vi "Build.vi"(9 "XYZTheta":dbl[](array[numeric]), 10 "Pattern Coordinates":dbl[][](array[numeric]), 11 "Crosshair Dispense in":refnum<class "Crosshair Dispense.lvclass">) -> (1 "Starting Coordinates":dbl[](array[numeric]), 3 "Crosshair Dispense out":refnum<class "Crosshair Dispense.lvclass">)   [LabVIEW 2019, in "Crosshair Dispense.lvclass"]
uses:
  Crosshair Dispense.lvclass
  Crosshair Dispense.lvclass/Crosshair Dispense.ctl
  <vilib>/Analysis/coordinate.llb/2D Cartesian Coordinate Rotation (Scalar).vi
  <vilib>/Analysis/NI_AALPro.lvlib
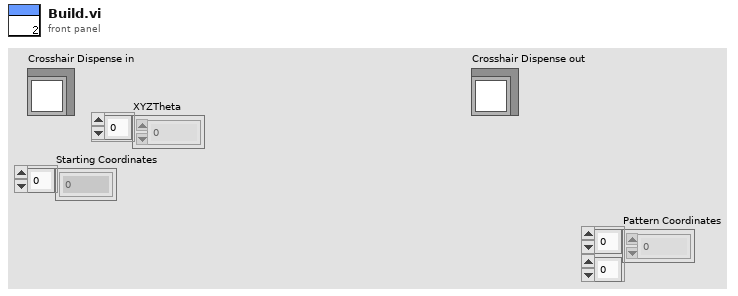
[diagram p1: front panel]
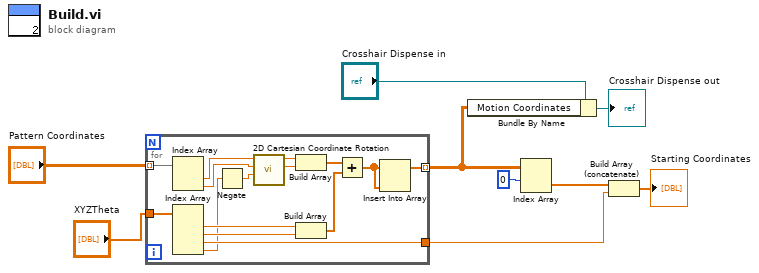
[diagram p0: block diagram]
diagram:
  n1 = for {
    tunnel: [w17] -> w6 mode=indexing
    tunnel: [w19] -> w7
    tunnel: "XYZTheta" -> [w14]
    tunnel: "Pattern Coordinates" -> [w12] mode=indexing
    n2 = Index Array(array=w12) -> (element #1=w11:dbl, element #2=w10:dbl)  [unwired: 2 in]
    n3 = Index Array(array=w14) -> (element #1=w22:dbl, element #2=w21:dbl, element #3=w19:dbl, element #4=w13:dbl)  [unwired: 4 in]
    n4 = Negate(x=w13) -> (-x=w16:dbl)
    n5 = call-poly <vilib>:"2D Cartesian Coordinate Rotation.vi"("theta"=w16, "y"=w10, "x"=w11) -> ("y out"=w24:dbl, "x out"=w23:dbl)  [unwired: 6 in, 1 out]
    n6 = Build Array(w23, w24) -> (w15:dbl[])
    n7 = Build Array(w22, w21) -> (w20:dbl[])
    n8 = Add(x=w15, y=w20) -> (x+y=w18:dbl[])
    n9 = Insert Into Array(array=w18, new element=w18) -> (w17:dbl[])  [unwired: 1 in]
  }
  n10 = Bundle By Name(cluster="Crosshair Dispense in", "Motion Coordinates"=w6) -> (→"Crosshair Dispense out":refnum<class "Crosshair Dispense.lvclass">)
  n11 = Index Array(array=w6, index (row)=0) -> (element=w4:dbl[])  [unwired: 1 in]
  n12 = Build Array (concatenate)(w4, w7) -> (→"Starting Coordinates":dbl[])
